vi "SineSum (1).vi"() -> ()   [LabVIEW 2018]
panel:
  out "Waveform Graph":cluster{dbl, "y":dbl, dbl[]}(graph)
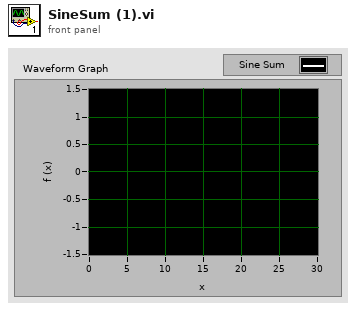
[diagram p1: front panel]
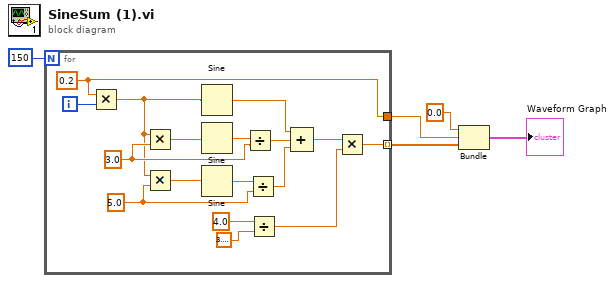
[diagram p0: block diagram]
diagram:
  n1 = for {
    N: 150 -> [_]
    tunnel: [w11] -> w2 mode=indexing
    tunnel: [w6] -> w3
    i -> [w22]
    w16 = 5.0 ("y")
    w18 = 3.0 ("y")
    w6 = 0.2 ("y")
    n2 = Multiply(x=w6, y=w22) -> (x*y=w7:dbl)
    n3 = Multiply(x=w7, y=w18) -> (x*y=w20:dbl)
    n4 = Multiply(x=w7, y=w16) -> (x*y=w21:dbl)
    n5 = Sine(x=w7) -> (sin(x)=w15:dbl)
    n6 = Sine(x=w20) -> (sin(x)=w19:dbl)
    n7 = Sine(x=w21) -> (sin(x)=w17:dbl)
    n8 = Divide(x=w19, y=w18) -> (x/y=w14:dbl)
    n9 = Divide(x=w17, y=w16) -> (x/y=w13:dbl)
    n10 = Divide(x=4.0, y=3.141592653589793) -> (x/y=w8:dbl)
    n11 = Compound Arithmetic op=ADD(w15, w14, w13) -> (w12:dbl)
    n12 = Multiply(x=w12, y=w8) -> (x*y=w11:dbl)
  }
  n13 = Bundle(0.0, "y"=w3, w2) -> (→"Waveform Graph":cluster{dbl, "y":dbl, dbl[]})  [unwired: 1 in]
